vi "Read Complete.vi"(8 "error in":errorcluster, 10 "connection ID":refnum<k16>, 11 "TeleOp Data Cluster in":T1) -> (0 "error out":errorcluster, 3 "TeleOp Data Cluster out":T1)   [LabVIEW 2018]
uses:
  TypeDefs/Teleop Data Cluster.ctl
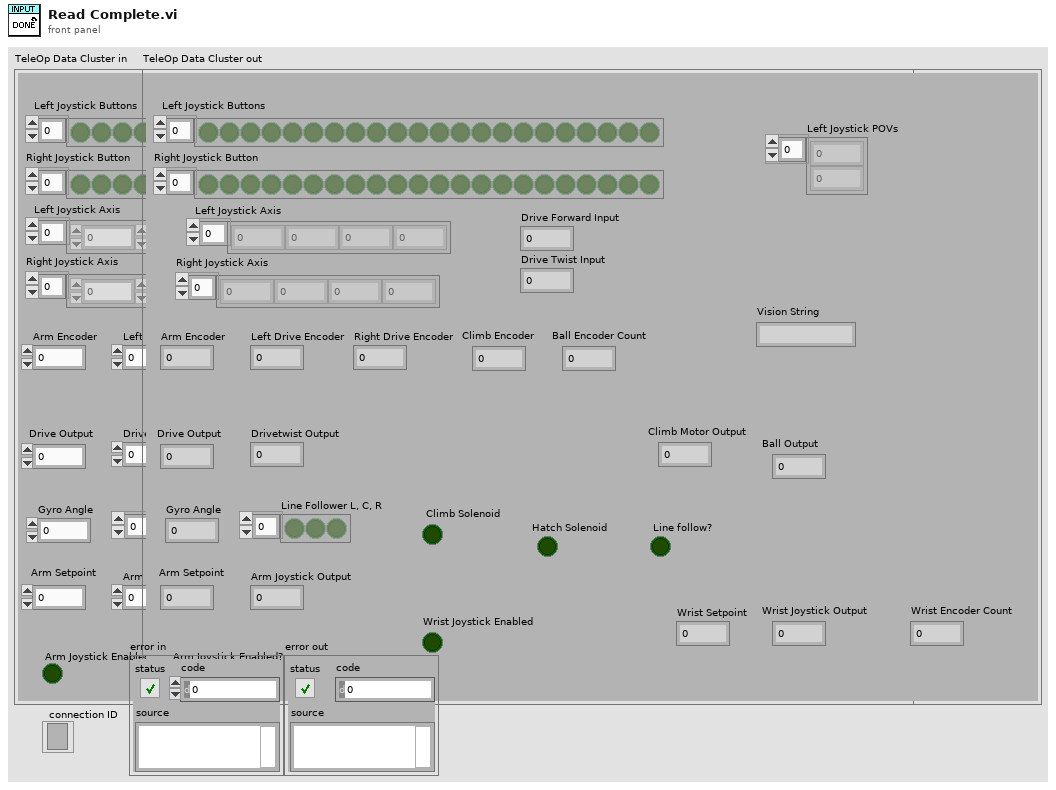
[diagram p1: front panel]
types:
  T1 = typedef "Teleop Data Cluster.ctl" = cluster{"Drive Forward Input ":dbl, "Drive Twist Input":dbl, "Drive Output":dbl, "Drivetwist Output":dbl, "Left Joystick Buttons":bool[], "Left Joystick Axis":dbl[], "Right Joystick Axis":dbl[], "Right Joystick Button":bool[], "Arm Encoder":dbl, "Left Drive Encoder":dbl, "Right Drive Encoder":dbl, "Gyro Angle ":dbl, "Arm Joystick Output  ":dbl, "Line Follower L, C, R ":bool[], "Line follow?":bool, " Climb Solenoid":bool, "Wrist Encoder Count":dbl, "Wrist Joystick Output":dbl, "Ball Encoder Count":dbl, "Ball Output":dbl, "Climb Encoder":dbl, "Climb Motor Output":dbl, " Hatch Solenoid":bool, "Arm Setpoint ":dbl, "Wrist Setpoint ":dbl, "Arm Joystick Enabled?":bool, "Wrist Joystick Enabled":bool, "Vision String":string, "Left Joystick POVs":i16[]}
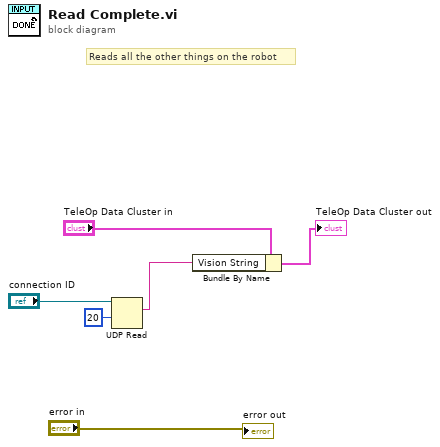
[diagram p0: block diagram]
diagram:
  # "Reads all the other things on the robot"
  n1 = UDP Read(connection ID="connection ID", timeout ms (25000)=20) -> (data out=w4:string)  [unwired: 2 in, 4 out]
  n2 = Bundle By Name(cluster="TeleOp Data Cluster in", "Vision String"=w4) -> (→"TeleOp Data Cluster out":T1)
  "error out" <- "error in"
